vi "Register For Events.vi"(8 "error in (no error)":errorcluster, 10 "Events To Register":T2[](array[typedef]), 11 "Session in":refnum<class "Plugin Session.lvclass">) -> (0 "error out":errorcluster, 2 "Event Refnum":T1, 3 "Session out":refnum<class "Plugin Session.lvclass">)   [LabVIEW 2021, in "InstrumentStudio Plugin SDK.lvlib" / "Plugin Session.lvclass"]
doc: "Call this VI to let the framework know which events you want to get notifications for. Only pass in events that you are going to handle in your event structure. There are four events available:\n\nShutdown\nThis event is fired when the document containing this VI is closing. The plugin must close all references and stop the VI. If the VI does not stop within a few seconds, the document will prompt the user to abort the running VI.\n\nProject Saved\nThis event is fired when the path of the Project changes. It passes event data for the updated project path and a Completion Id. The plugin must call Notify Event Complete with this Completion Id to let the framework know its processing is complete. Failure to do this will result in a hang.\n\nStop All Outputs\nThe Stop All Outputs event is fired when the 'Stop all outputs' button is pressed on the document toolbar. It notifies the plugin that it should cease sending output data to any external devices.\n\nGeneric Message\nReserved for internal/future use by InstrumentStudio.\n\nActive Pin Map Changed\nThis event is fired when either the active pin map changes or the contents of the active pin map change. It notifies the plugin that it should make any updates to UI elements that depend on the pin map.\n\nSelected Sites Changed\nThis event is fired when the selected sites in the document toolbar changes. It notifies the plugin that it should make any updates that depend on which sites should be displayed."
uses:
  Plugin Session.lvclass
  Plugin Events Enum.ctl
  Event Registration Refnum.ctl
  Plugin Events.ctl
  Plugin Session.lvclass/Plugin Session.ctl
  Read Session Id.vi
  Read Plugin Events.vi
  Read Event Refnum.vi
  InstrumentStudio Plugin SDK.lvlib
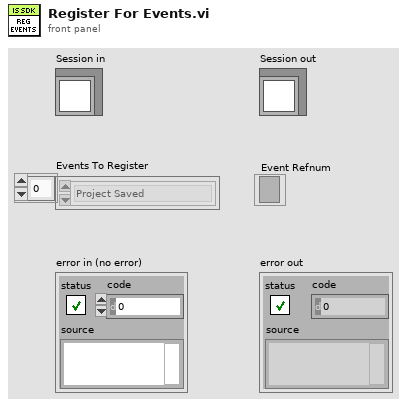
[diagram p1: front panel]
types:
  T1 = typedef "InstrumentStudio Plugin SDK.lvlib/Event Registration Refnum.ctl" = refnum<event-registration>
  T2 = typedef "InstrumentStudio Plugin SDK.lvlib/Plugin Events Enum.ctl" = enum32{"Shutdown", "Project Saved", "Stop All Outputs", "Generic Message", "Active Pin Map Changed", "Selected Sites Changed"}
  T3 = typedef "InstrumentStudio Plugin SDK.lvlib/Plugin Events.ctl" = cluster{"Shutdown":refnum<user-event>, "Project Saved":refnum<user-event>, "Stop All Outputs":refnum<user-event>, "Generic Message":refnum<user-event>, "Active Pin Map Changed":refnum<user-event>, "Selected Sites Changed":refnum<user-event>}
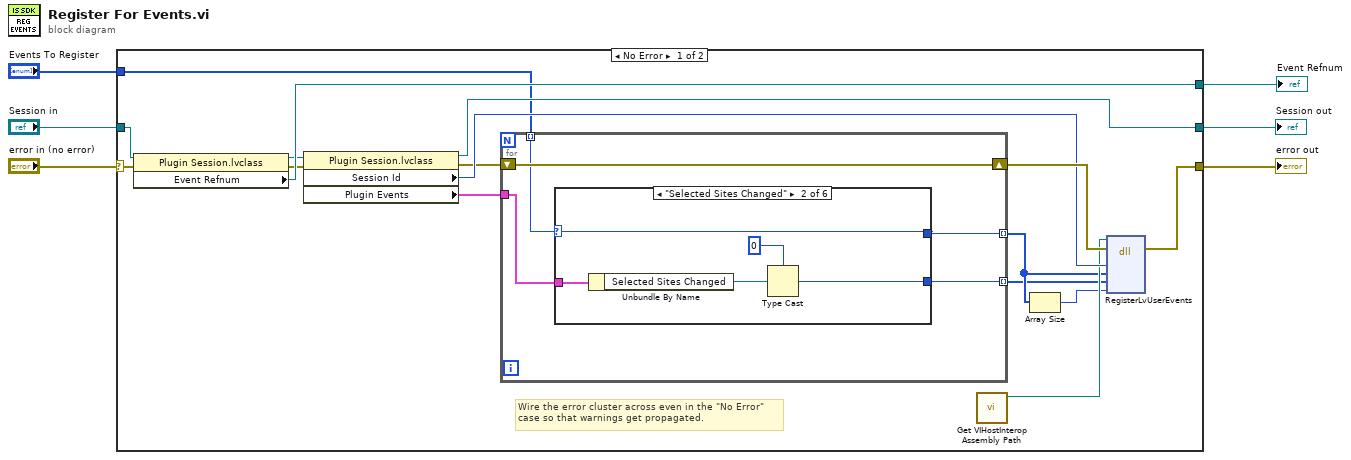
[diagram p0: block diagram]
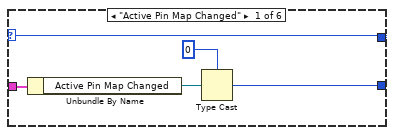
[diagram p2: hidden frame]
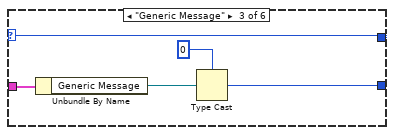
[diagram p3: hidden frame]
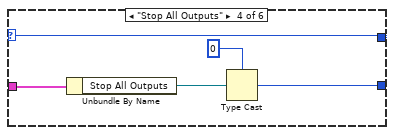
[diagram p4: hidden frame]
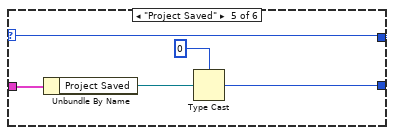
[diagram p5: hidden frame]
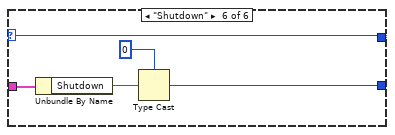
[diagram p6: hidden frame]
diagram:
  n1 = case shown="No Error" "error in (no error)" {
    selector: "error in (no error)" -> [w21 w59]
    tunnel: [w19 w59] -> w5
    tunnel: [w15 w58] -> w3
    tunnel: "Session in" -> [w22 w58]
    tunnel: "Events To Register" -> [w11 _]
    tunnel: [w18 _] -> w1
    frame No Error {
      # "Wire the error cluster across even in the \"No Error\"\ncase so that warnings get propagated."
      n2 = property class="Plugin Session.lvclass"(reference=w22, error in=w21) -> (reference out=w16:refnum<class "Plugin Session.lvclass">, error out=w17:errorcluster, "Event Refnum"=w18:T1)
      n3 = property class="Plugin Session.lvclass"(reference=w16, error in=w17) -> (reference out=w15:refnum<class "Plugin Session.lvclass">, error out=w12:errorcluster, "Session Id"=w14:u64, "Plugin Events"=w13:T3)
      n4 = for {
        shift-right: [w26] -> w20
        shift-left: w12 -> [w26]
        tunnel: w13 -> [w27]
        tunnel: w11 -> [w25] mode=indexing
        tunnel: [w24] -> w9 mode=indexing
        tunnel: [w23] -> w7 mode=indexing
        n5 = case shown="\"Selected Sites Changed\"" w25 {
          selector: w25 -> [w28 w33 w38 w43 w48 w53]
          tunnel: [w30 w35 w40 w45 w50 w55] -> w23
          tunnel: w27 -> [w29 w34 w39 w44 w49 w54]
          tunnel: [w28 w33 w38 w43 w48 w53] -> w24
          frame "Active Pin Map Changed" {
            n6 = Unbundle By Name(w29) -> ("Active Pin Map Changed"=w32:refnum<user-event>)
            n7 = Type Cast(type=u32 0, x=w32) -> (*(type *) &x=w30:u32)
          }
          frame "Selected Sites Changed" {
            n8 = Unbundle By Name(w34) -> ("Selected Sites Changed"=w37:refnum<user-event>)
            n9 = Type Cast(type=u32 0, x=w37) -> (*(type *) &x=w35:u32)
          }
          frame "Generic Message" {
            n10 = Unbundle By Name(w39) -> ("Generic Message"=w42:refnum<user-event>)
            n11 = Type Cast(type=u32 0, x=w42) -> (*(type *) &x=w40:u32)
          }
          frame "Stop All Outputs" {
            n12 = Unbundle By Name(w44) -> ("Stop All Outputs"=w47:refnum<user-event>)
            n13 = Type Cast(type=u32 0, x=w47) -> (*(type *) &x=w45:u32)
          }
          frame "Project Saved" {
            n14 = Unbundle By Name(w49) -> ("Project Saved"=w52:refnum<user-event>)
            n15 = Type Cast(type=u32 0, x=w52) -> (*(type *) &x=w50:u32)
          }
          frame "Shutdown" {
            n16 = Unbundle By Name(w54) -> ("Shutdown"=w57:refnum<user-event>)
            n17 = Type Cast(type=u32 0, x=w57) -> (*(type *) &x=w55:u32)
          }
        }
      }
      n18 = call "Get VIHostInterop Assembly Path.vi"() -> ("VIHost.Interop Assembly"=w10:path)  [unwired: 11 in]
      n19 = Array Size(array=w9) -> (size(s)=w8:i32)
      n20 = dll-call lib="C:/ASW/Source/InstrumentStudio/IFDistribution/VIHostPanel/objects/export/targets/win64U/x64/msvc-14.0/debug/NationalInstruments.VIHost.Interop.dll" fn="RegisterLvUserEvents"(path in=w10, error in=w20, "hostId"=w14, "eventIds"=w9, "eventRefs"=w7, "numElements"=w8) -> (error out=w19:errorcluster)  [unwired: 6 in, 1 out]
    }
    frame Error {
    }
  }
  "error out" <- w5
  "Session out" <- w3
  "Event Refnum" <- w1
